vi "search_array_for_limit.vi"(4 "Window Size":dbl, 6 "Reference Time":dbl, 9 "Step Size":i32, 10 "Start Index":i32, 11 "Times":dbl[](array[numeric])) -> (1 "Valid":bool, 2 "End Index":i32, 3 "Times out":dbl[](array[numeric]))   [LabVIEW 2025, in "LabJackEKG.lvlib"]
uses:
  LabJackEKG.lvlib
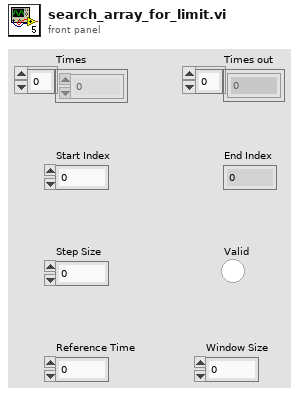
[diagram p1: front panel]
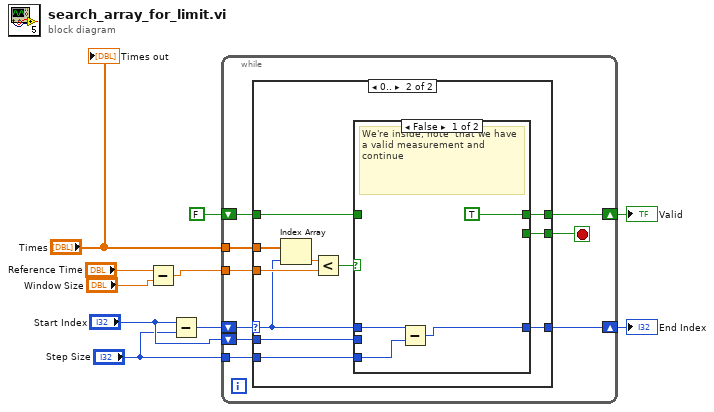
[diagram p0: block diagram]
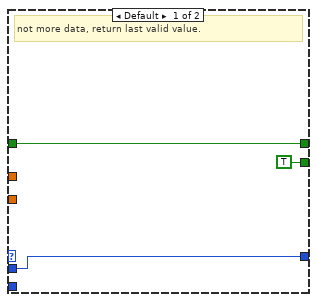
[diagram p2: hidden frame]
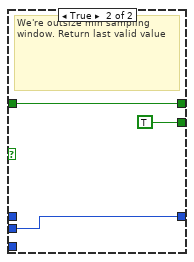
[diagram p3: hidden frame]
diagram:
  n1 = Subtract(x="Reference Time", y="Window Size") -> (x-y=w2:dbl)
  n2 = Subtract(x="Start Index", y="Step Size") -> (x-y=w9:i32)
  n3 = while {
    tunnel: w2 -> [w19]
    shift-right: [w11] -> w3
    shift-left: w9 -> [w18]
    tunnel: "Times" -> [w17]
    shift-right: [w14] -> w4
    shift-left: FALSE -> [w15]
    tunnel: "Step Size" -> [w16]
    shift-left: "Start Index" -> [w13]
    stop <- w12 stop-if-true
    n4 = case shown="0.." w18 {
      selector: w18 -> [_ w29]
      tunnel: w19 -> [_ w33]
      tunnel: w17 -> [_ w32]
      tunnel: w16 -> [_ w30]
      tunnel: w15 -> [w20 w27]
      tunnel: [w20 w26] -> w14
      tunnel: w13 -> [w22 w24]
      tunnel: [w22 w25] -> w11
      tunnel: [TRUE w23] -> w12
      frame Default {
        # "not more data, return last valid value."
      }
      frame 0.. {
        n5 = Index Array(array=w32, index=w29) -> (element=w31:dbl)
        n6 = Less?(x=w31, y=w33) -> (x < y?=w28:bool)
        n7 = case shown="False" w28 {
          tunnel: w30 -> [w36 _]
          tunnel: w29 -> [w37 _]
          tunnel: w27 -> [_ w40]
          tunnel: [TRUE w40] -> w26
          tunnel: [w34 w39] -> w25
          tunnel: w24 -> [_ w39]
          tunnel: [_ TRUE] -> w23
          frame False {
            # "We're inside, note  that we have a valid measurement and continue"
            n8 = Subtract(x=w37, y=w36) -> (x-y=w34:i32)
          }
          frame True {
            # "We're outsize min sampling window. Return last valid value"
          }
        }
      }
    }
  }
  "Valid" <- w4
  "End Index" <- w3
  "Times out" <- "Times"
